vi "ShootGridPoint.vi"(0 "object in":refnum<class "Map.lvclass">, 2 "GridPoint":T1, 5 "error in (no error)":errorcluster) -> (14 "object out":refnum<class "Map.lvclass">, 16 "Hit?":bool, 17 "Sunk?":bool, 19 "error out":errorcluster)   [LabVIEW 2015, in "Map.lvclass"]
doc: "Shoots at a grid position on the map and returns if the shot was a hit and if a ship was sunk."
uses:
  Map.lvclass
  TypDefs/Coordinates.ctl
  Map.lvclass/Map.ctl
  TypDefs/GridState.ctl
  Battleship_class/Battleship.lvclass
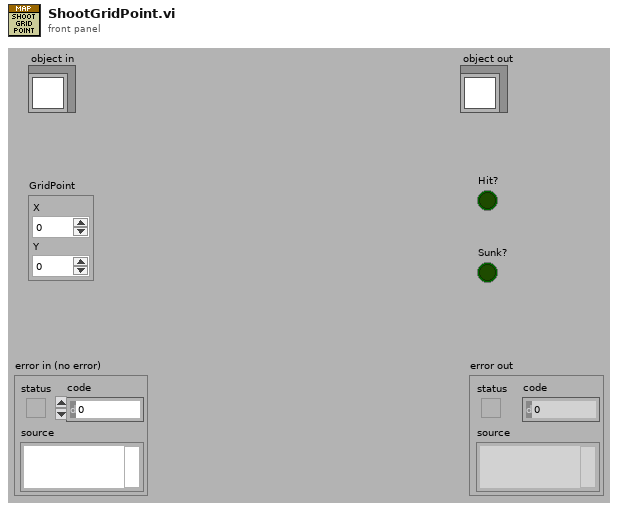
[diagram p1: front panel]
types:
  T1 = typedef "Coordinates.ctl" = cluster{"X":i32, "Y":i32}
  T2 = typedef "GridState.ctl" = enum16{"Sea", "Ship", "Hit", "Miss"}
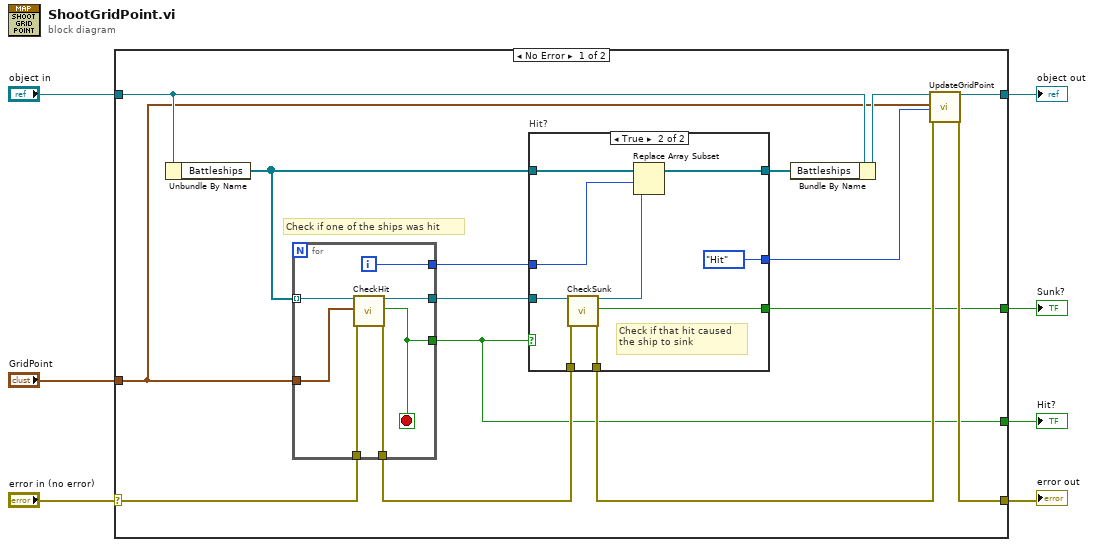
[diagram p0: block diagram]
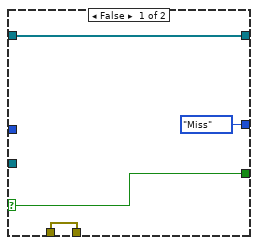
[diagram p2: hidden frame]
diagram:
  n1 = case shown="No Error" "error in (no error)" {
    selector: "error in (no error)" -> [w22 w44]
    tunnel: [w21 w44] -> w6
    tunnel: [w19 w43] -> w4
    tunnel: "object in" -> [w20 w43]
    tunnel: "GridPoint" -> [w9 _]
    tunnel: [w8 _] -> w1
    tunnel: [w15 _] -> w2
    frame No Error {
      # "Check if one of the ships was hit"
      n2 = Unbundle By Name(w20) -> ("Battleships"=w12:refnum<class "Battleship.lvclass">[])
      n3 = for {
        tunnel: w12 -> [w42] mode=indexing
        tunnel: w9 -> [w41]
        tunnel: [w40] -> w8
        tunnel: w22 -> [w39]
        tunnel: [w38] -> w16
        tunnel: [w37] -> w18
        tunnel: [w36] -> w11
        i -> [w36]
        stop <- w40 stop-if-true
        n4 = call-dynamic "CheckHit.vi"("object in"=w42, "Shot\nCoordinates"=w41, "error in (no error)"=w39) -> ("object out"=w37:refnum<class "Battleship.lvclass">, "Hit?"=w40:bool, "error out"=w38:errorcluster)  [unwired: 14 in]
      }
      n5 = case "Hit?" shown="True" w8 {
        selector: w8 -> [w23 _]
        tunnel: w18 -> [_ w35]
        tunnel: [w25 w34] -> w17
        tunnel: w16 -> [w25 w33]
        tunnel: [w23 w32] -> w15
        tunnel: [w26 w31] -> w13
        tunnel: w12 -> [w26 w30]
        tunnel: w11 -> [_ w28]
        tunnel: [GridState."Miss" ("State") GridState."Hit" ("State")] -> w10
        frame False {
        }
        frame True {
          # "Check if that hit caused\nthe ship to sink"
          n6 = call-dynamic "CheckSunk.vi"("object in"=w35, "error in (no error)"=w33) -> ("object out"=w29:refnum<class "Battleship.lvclass">, "Sunk?"=w32:bool, "error out"=w34:errorcluster)  [unwired: 15 in]
          n7 = Replace Array Subset(array=w30, new element=w29, index=w28) -> (w31:refnum<class "Battleship.lvclass">[])
        }
      }
      n8 = Bundle By Name(cluster=w20, "Battleships"=w13) -> (w14:refnum<class "Map.lvclass">)
      n9 = call-dynamic "UpdateGridPoint.vi"("object in"=w14, "Coordinates"=w9, "State"=w10, "error in (no error)"=w17) -> ("object out"=w19:refnum<class "Map.lvclass">, "error out"=w21:errorcluster)  [unwired: 13 in, 1 out]
    }
    frame Error {
    }
  }
  "error out" <- w6
  "object out" <- w4
  "Sunk?" <- w2
  "Hit?" <- w1
